vi "Keithley 2400 - VoltReadSource.vi"(0 "error in (no error)":errorcluster, 7 "Tensão aplicada:":dbl=10.0, 11 "Porta:":refnum<visa-resource-name>="COM5") -> (2 "Corrente:":dbl, 3 "Tensão:":dbl, 8 "error out":errorcluster)   [LabVIEW 2017]
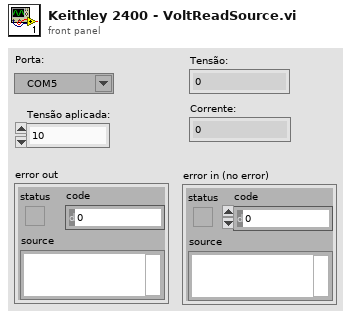
[diagram p1: front panel]
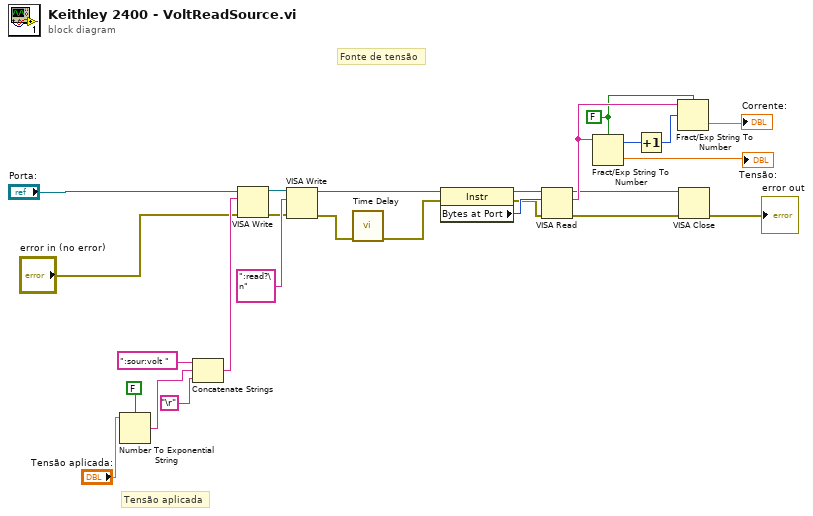
[diagram p0: block diagram]
diagram:
  w8 = FALSE ("use system decimal point (T)")
  # "Tensão aplicada"
  # "Fonte de tensão"
  n1 = Number To Exponential String(number="Tensão aplicada:", 1:FALSE ("use system decimal point (T)")) -> (E-format string=w7:string)  [unwired: 2 in]
  n2 = Concatenate Strings(":sour:volt " ("string"), w7, "\r") -> (w25:string)
  n3 = VISA Write(VISA resource name="Porta:", write buffer=w25, error in (no error)="error in (no error)") -> (VISA resource name out=w21:refnum<visa-resource-name>, error out=w22:errorcluster)  [unwired: 1 out]
  n4 = VISA Write(VISA resource name=w21, write buffer=":read?\n", error in (no error)=w22) -> (VISA resource name out=w19:refnum<visa-resource-name>, error out=w23:errorcluster)  [unwired: 1 out]
  n5 = call "Time Delay"("error in (no error)"=w23) -> ("error out"=w20:errorcluster)  [unwired: 10 in]
  n6 = property class="Instr"(reference=w19, error in=w20) -> (reference out=w17:refnum<visa-resource-name>, error out=w16:errorcluster, "Bytes at Port"=w18:u32)
  n7 = VISA Read(VISA resource name=w17, byte count=w18, error in (no error)=w16) -> (VISA resource name out=w2:refnum<visa-resource-name>, read buffer=w13:string, error out=w3:errorcluster)  [unwired: 1 out]
  n8 = Fract/Exp String To Number(use system decimal point (T)=w8, string=w13) -> (offset past number=w12:i32, number=→"Tensão:":dbl)  [unwired: 2 in]
  n9 = Increment(x=w12) -> (x+1=w11:i32)
  n10 = Fract/Exp String To Number(use system decimal point (T)=w8, string=w13, offset=w11) -> (number=→"Corrente:":dbl)  [unwired: 1 in, 1 out]
  n11 = VISA Close(VISA resource name=w2, error in (no error)=w3) -> (error out=→"error out":errorcluster)
